vi "Strip Method Name.vi"(11 "Full Qualified Name in":string) -> (3 "Plain Method Name out":string)   [LabVIEW 2020, in "Peek Window.lvlib"]
uses:
  Peek Window.lvlib
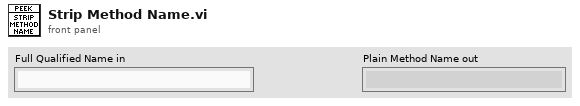
[diagram p1: front panel]
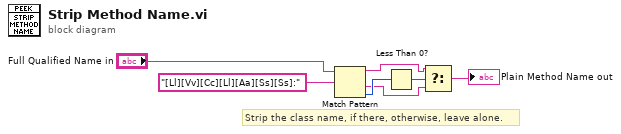
[diagram p0: block diagram]
diagram:
  # "Strip the class name, if there, otherwise, leave alone."
  n1 = Match Pattern(string="Full Qualified Name in", regular expression="[Ll][Vv][Cc][Ll][Aa][Ss][Ss]:") -> (before substring=w2:string, after substring=w1:string, offset past match=w4:i32)  [unwired: 1 in, 1 out]
  n2 = Less Than 0?(x=w4) -> (x < 0?=w3:bool)
  n3 = Select(t=w2, s=w3, f=w1) -> (s? t:f=→"Plain Method Name out":string)
